vi "Get Game Board.vi"(11 "Game Board in":refnum<class "Game Board.lvclass">) -> (2 "Game Board":u32[][](array[colorbox]))   [LabVIEW 2015, in "Game Board.lvclass"]
uses:
  Game Board.lvclass
  Game Board.lvclass/Game Board.ctl
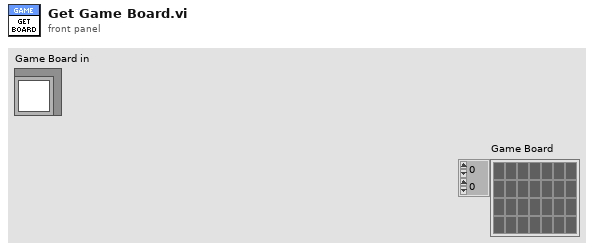
[diagram p1: front panel]
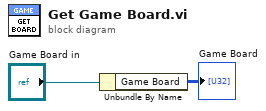
[diagram p0: block diagram]
diagram:
  n1 = Unbundle By Name("Game Board in") -> ("Game Board"=→"Game Board":u32[][])
